vi "FROG_TraceOverlay.vi"(4 "Experiment Trace":dbl[][](array[numeric]), 5 "Complex Electric Field":cdb[][](array[numeric])) -> (2 "Overlayed Complex Electric Field":cdb[][](array[numeric]))   [LabVIEW 2013]
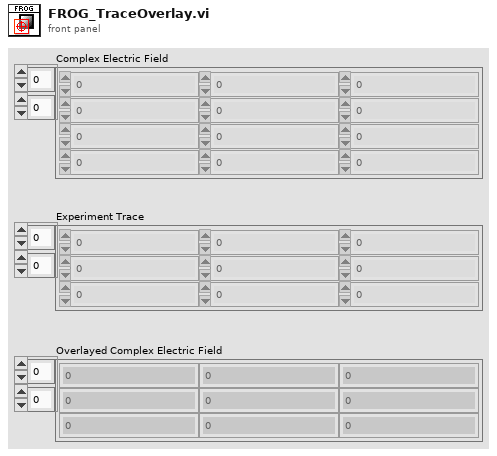
[diagram p1: front panel]
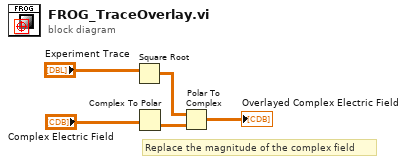
[diagram p0: block diagram]
diagram:
  # "Replace the magnitude of the complex field"
  n1 = Square Root ("Square Root.vi")(x="Experiment Trace") -> (sqrt(x)=w4:dbl[][])
  n2 = Complex To Polar(r * e^(i*theta)="Complex Electric Field") -> (theta=w5:dbl[][])  [unwired: 1 out]
  n3 = Polar To Complex(1:w5, 2:w4) -> (0:→"Overlayed Complex Electric Field":cdb[][])
